vi "Update Value.vi"(8 "error in (no error)":errorcluster, 11 "GUI Element in":refnum<class "GUI Element.lvclass">) -> (0 "error out":errorcluster, 2 "Value":variant, 3 "GUI Element out":refnum<class "GUI Element.lvclass">)   [LabVIEW 2020, in "VolatusGUI.lvlib" / "GUI Element.lvclass"]
uses:
  GUI Element.lvclass
  GUI Element.lvclass/GUI Element.ctl
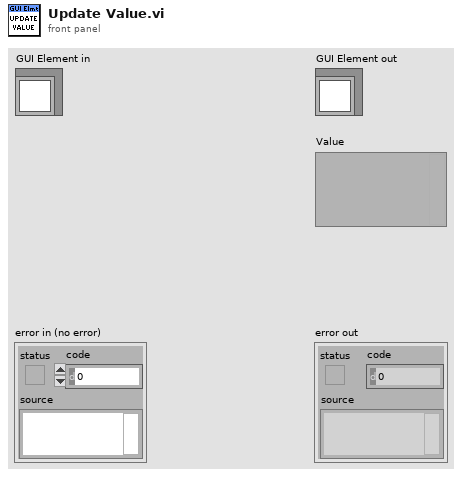
[diagram p1: front panel]
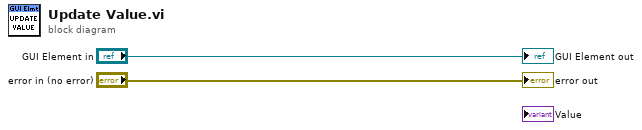
[diagram p0: block diagram]
diagram:
  "error out" <- "error in (no error)"
  "GUI Element out" <- "GUI Element in"
